vi "camara 2.vi"() -> ()   [LabVIEW 2010]
uses:
  <vilib>/addons/PixeLINK/Low Level Functions/CAMERA_FEATURES.llb/TDPU-CameraFeatures-PixelFormat.ctl
  <vilib>/addons/PixeLINK/Low Level Functions/ACQUISITION.llb/TDPU-Acquisition-StreamState.ctl
  <vilib>/addons/PixeLINK/Low Level Functions/CAMERA_FEATURES.llb/TDPU-CameraFeatures-FeatureIds.ctl
  <vilib>/addons/PixeLINK/Low Level Functions/CAMERA_FEATURES.llb/TDPU-CameraFeatures-FeatureFlags.ctl
panel:
  out "Data OUT":u8[](array[numeric])
  in  "Streeam":bool
  in  "Pixel Format Requerido":T1 items=["PIXEL_FORMAT_MONO8", "PIXEL_FORMAT_MONO16", "PIXEL_FORMAT_YUV422", "PIXEL_FORMAT_BAYER8_GRBG", "PIXEL_FORMAT_BAYER16_GRBG", "PIXEL_FORMAT_RGB24", "PIXEL_FORMAT_RGB48", "PIXEL_FORMAT_BAYER8_RGGB", "PIXEL_FORMAT_BAYER8_GBRG ", "PIXEL_FORMAT_BAYER8_BGGR ", "PIXEL_FORMAT_BAYER16_RGGB ", "PIXEL_FORMAT_BAYER16_GBRG", "PIXEL_FORMAT_BAYER16_BGGR", "PIXEL_FORMAT_RGB32"]
  out "Numeric":i32
  in  "Stop App":bool
  out "Numero de Camaras":u32
  in  "Selector":u16(ring) items=["776002034"]
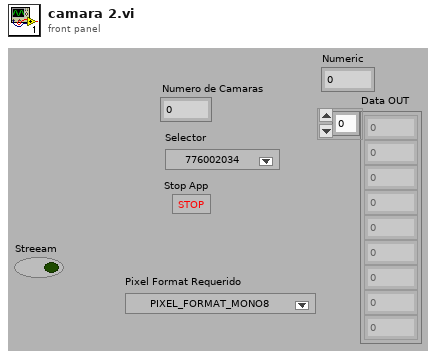
[diagram p1: front panel]
types:
  T1 = typedef "TDPU-CameraFeatures-PixelFormat.ctl" = u16
  T2 = typedef "TDPU-Acquisition-StreamState.ctl" = u32
  T3 = typedef "TDPU-CameraFeatures-FeatureIds.ctl" = u32
  T4 = typedef "TDPU-CameraFeatures-FeatureFlags.ctl" = u32
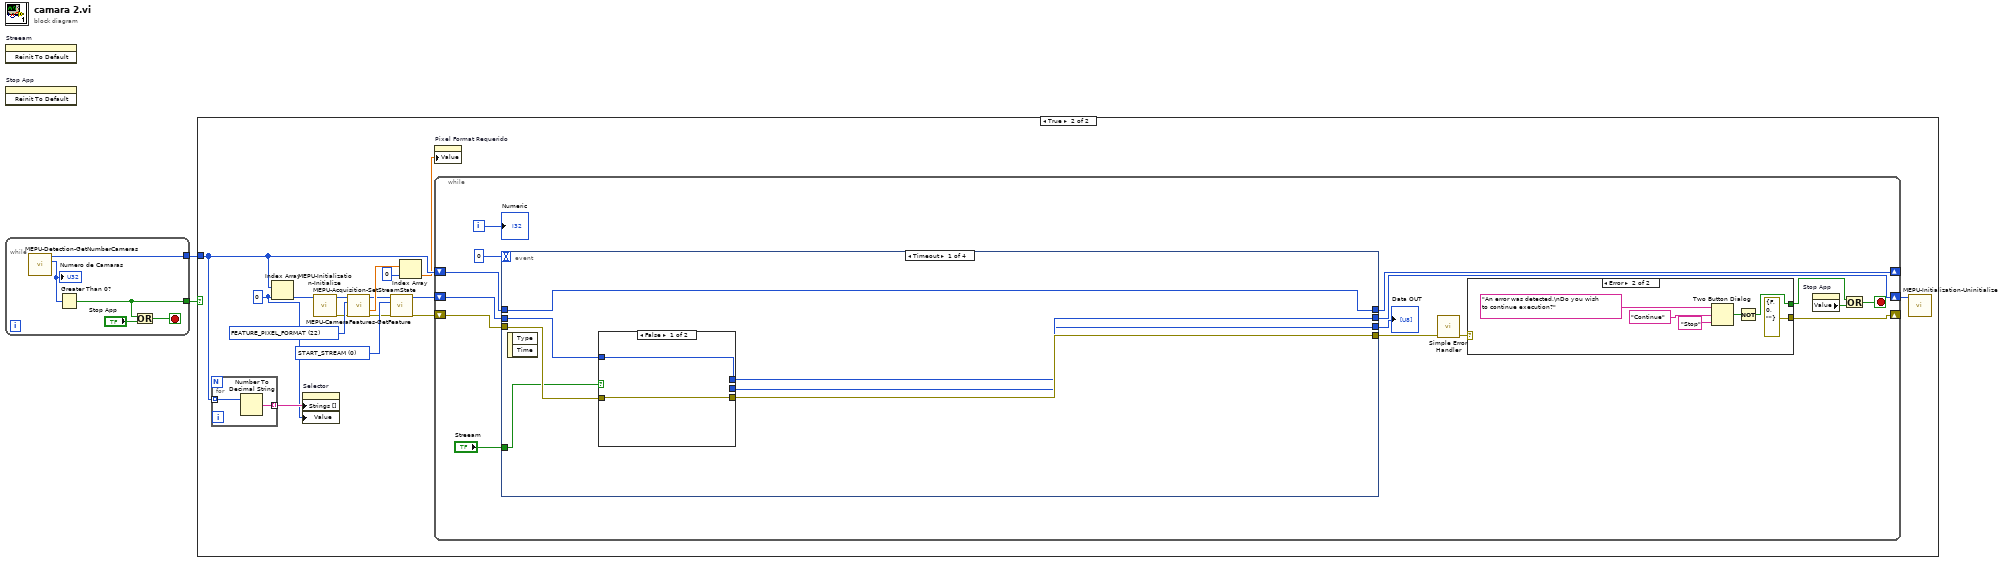
[diagram p0: block diagram]
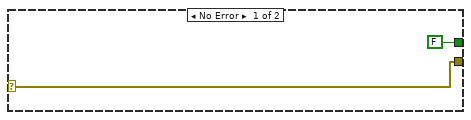
[diagram p3: hidden frame]
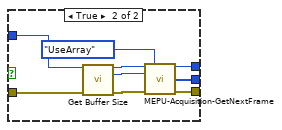
[diagram p4: hidden frame]
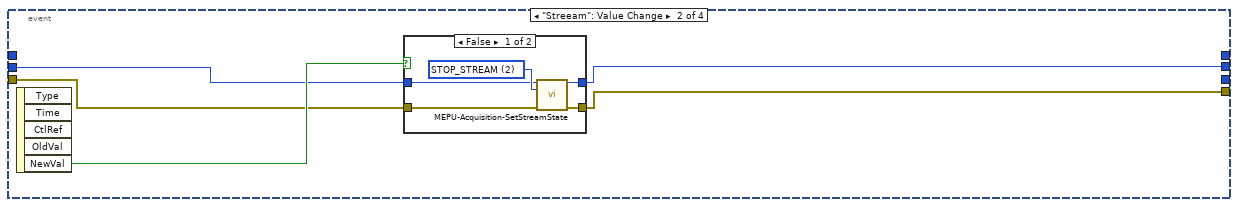
[diagram p5: hidden frame]
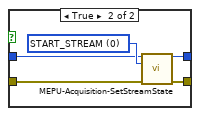
[diagram p6: hidden frame]
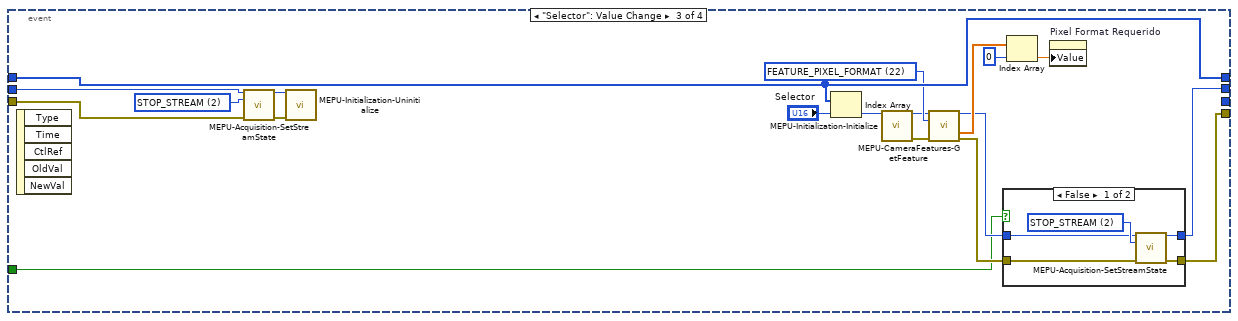
[diagram p7: hidden frame]
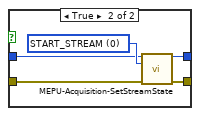
[diagram p8: hidden frame]
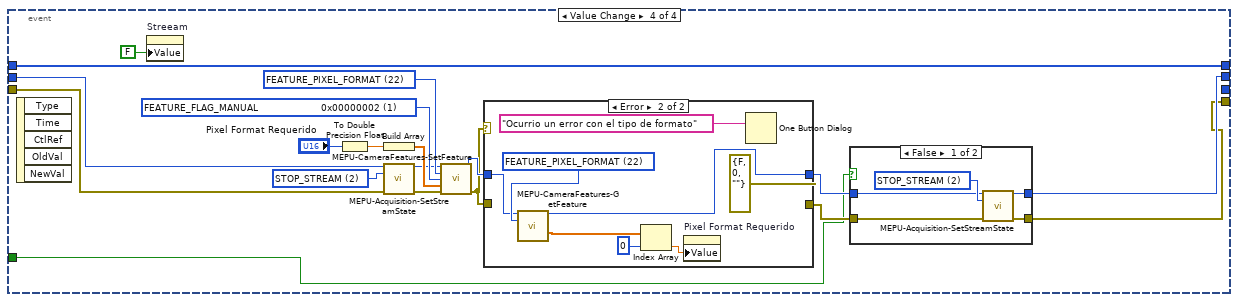
[diagram p9: hidden frame]
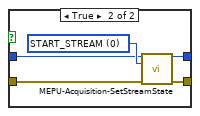
[diagram p10: hidden frame]
diagram:
  n1 = invoke on="Streeam" class="Bool (strict)" method="Reinit To Default"() -> ()  [unwired: 3 in, 3 out]
  n2 = invoke on="Stop App" class="Bool (strict)" method="Reinit To Default"() -> ()  [unwired: 3 in, 3 out]
  n3 = while {
    tunnel: [w7] -> w2
    tunnel: [w3] -> w1
    stop <- w5 stop-if-true
    n4 = call <vilib>:"MEPU-Detection-GetNumberCameras.vi"() -> ("LV_SerialNumbers OUT"=w7:u32[], "LV_NumberSerial OUT"=w4:u32)  [unwired: 13 in, 1 out]
    "Numero de Camaras" <- w4
    n5 = Greater Than 0?(x=w4) -> (x > 0?=w3:bool)
    n6 = Or(x=w3, y="Stop App") -> (x .or. y?=w5:bool)
  }
  n7 = case shown="True" w1 {
    tunnel: w2 -> [_ w21]
    frame False {
    }
    frame True {
      w12 = T2 0 items=["START_STREAM", "PAUSE_STREAM", "STOP_STREAM"] ("uStreamState IN")
      w17 = T3 22 items=["FEATURE_BRIGHTNESS", "FEATURE_EXPOSURE", "FEATURE_SHARPNESS", "FEATURE_WHITE_BAL", "FEATURE_HUE", "FEATURE_SATURATION", "FEATURE_GAMMA", "FEATURE_SHUTTER", "FEATURE_GAIN", "FEATURE_IRIS", "FEATURE_FOCUS", "FEATURE_TEMPERATURE", "FEATURE_TRIGGER", "FEATURE_ZOOM", "FEATURE_PAN", "FEATURE_TILT", "FEATURE_OPT_FILTER", "FEATURE_GPIO", "FEATURE_FRAME_RATE", "FEATURE_ROI", "FEATURE_FLIP", "FEATURE_PIXEL_ADDRESSING", "FEATURE_PIXEL_FORMAT", "FEATURE_EXTENDED_SHUTTER", "FEATURE_AUTO_ROI", "FEATURE_LOOKUP_TABLE", "FEATURE_MEMORY_CHANNEL", "FEATURE_WHITE_SHADING", "FEATURE_ROTATE", "FEATURE_IMAGER_CLK_DIVISOR", "FEATURE_TRIG_WITH_CNTRLD_LIGHT", "FEATURE_MAX_PIXEL_SIZE"] ("uFeatureId IN")
      w20 = 0
      n8 = for {
        tunnel: w21 -> [w149] mode=indexing
        tunnel: [w148] -> w23 mode=indexing
        n9 = Number To Decimal String(number=w149) -> (decimal integer string=w148:string)  [unwired: 1 in]
      }
      n10 = Index Array(array=w21, index=w20) -> (element=w22:u32)
      n11 = property on="Selector" class="Ring (strict)"("Strings []"=w23, "Value"=w20) -> ()  [unwired: 2 in, 2 out]
      n12 = call <vilib>:"MEPU-Initialization-Initialize.vi"("uSerialNumber IN"=w22) -> ("phCamera OUT"=w14:u32, "Error OUT"=w13:errorcluster)  [unwired: 12 in, 1 out]
      n13 = call <vilib>:"MEPU-CameraFeatures-GetFeature.vi"("hCamera IN"=w14, "uFeatureId IN"=w17, "Error IN"=w13) -> ("hCamera OUT"=w9:u32, "pParms OUT"=w18:dbl[], "Error OUT"=w10:errorcluster)  [unwired: 8 in, 2 out]
      n14 = call <vilib>:"MEPU-Acquisition-SetStreamState.vi"("hCamera IN"=w9, "uStreamState IN"=w12, "Error IN"=w10) -> ("hCamera OUT"=w8:u32, "Error OUT"=w11:errorcluster)  [unwired: 11 in]
      n15 = Index Array(array=w18, index=0) -> (element=w15:dbl)
      n16 = property on="Pixel Format Requerido" class="Ring (strict)"("Value"=w15) -> ()  [unwired: 2 in, 2 out]
      n17 = while {
        shift-right: [w37] -> _
        shift-left: w21 -> [w38]
        shift-right: [w26] -> w19
        shift-left: w8 -> [w36]
        shift-right: [w31] -> _
        shift-left: w11 -> [w35]
        i -> [w30]
        stop <- w32 stop-if-true
        n18 = event shown="[0] Timeout" {
          selector: _ -> [_ _ _ _]
          dyn-events: _ -> [_ _ _ _]
          timeout: 0 -> [_ _ _ _]
          tunnel: w38 -> [w53 _ w96 w114]
          tunnel: [w50 w66 w81 w113] -> w26
          tunnel: [w51 w65 w84 w112] -> w27
          tunnel: [w53 _ w96 w114] -> w37
          tunnel: w36 -> [w52 w68 w85 w120]
          tunnel: w35 -> [w48 w67 w86 w119]
          tunnel: [w49 _ _ _] -> w25
          tunnel: "Streeam" -> [w47 _ w80 w109]
          event Timeout {
            n19 = event-data() -> ()  [unwired: 1 in, 2 out]
            n20 = case shown="False" w47 {
              tunnel: w52 -> [w55 w60]
              tunnel: [w54 w59] -> w51
              tunnel: [w55 w58] -> w50
              tunnel: [_ w57] -> w49
              tunnel: w48 -> [w54 w56]
              frame False {
              }
              frame True {
                n21 = call "Get Buffer Size.vi"("phCamera IN"=w60, "Error IN"=w56) -> ("phCamera OUT"=w61:u32, "uBufferSize OUT"=w63:u32, "Error OUT"=w64:errorcluster)  [unwired: 11 out]
                n22 = call <vilib>:"MEPU-Acquisition-GetNextFrame.vi"("hCamera IN"=w61, "Mode IN"=enum16{"UseArray", "UsePointer"}."UseArray", "uBufferSize IN"=w63, "Error IN"=w64) -> ("hCamera OUT"=w58:u32, "Data OUT"=w57:u8[], "Error OUT"=w59:errorcluster)  [unwired: 7 in, 2 out]
              }
            }
          }
          event "Streeam": Value Change {
            n23 = event-data() -> ("NewVal"=w69:bool)  [unwired: 1 in, 4 out]
            n24 = case shown="False" w69 {
              tunnel: w68 -> [w73 w78]
              tunnel: w67 -> [w72 w77]
              tunnel: [w70 w76] -> w65
              tunnel: [w71 w75] -> w66
              frame False {
                w74 = T2 2 items=["START_STREAM", "PAUSE_STREAM", "STOP_STREAM"] ("uStreamState IN")
                n25 = call <vilib>:"MEPU-Acquisition-SetStreamState.vi"("hCamera IN"=w73, "uStreamState IN"=w74, "Error IN"=w72) -> ("hCamera OUT"=w71:u32, "Error OUT"=w70:errorcluster)  [unwired: 11 in]
              }
              frame True {
                w79 = T2 0 items=["START_STREAM", "PAUSE_STREAM", "STOP_STREAM"] ("uStreamState IN")
                n26 = call <vilib>:"MEPU-Acquisition-SetStreamState.vi"("hCamera IN"=w78, "uStreamState IN"=w79, "Error IN"=w77) -> ("hCamera OUT"=w75:u32, "Error OUT"=w76:errorcluster)  [unwired: 11 in]
              }
            }
          }
          event "Selector": Value Change {
            w89 = T2 2 items=["START_STREAM", "PAUSE_STREAM", "STOP_STREAM"] ("uStreamState IN")
            w95 = T3 22 items=["FEATURE_BRIGHTNESS", "FEATURE_EXPOSURE", "FEATURE_SHARPNESS", "FEATURE_WHITE_BAL", "FEATURE_HUE", "FEATURE_SATURATION", "FEATURE_GAMMA", "FEATURE_SHUTTER", "FEATURE_GAIN", "FEATURE_IRIS", "FEATURE_FOCUS", "FEATURE_TEMPERATURE", "FEATURE_TRIGGER", "FEATURE_ZOOM", "FEATURE_PAN", "FEATURE_TILT", "FEATURE_OPT_FILTER", "FEATURE_GPIO", "FEATURE_FRAME_RATE", "FEATURE_ROI", "FEATURE_FLIP", "FEATURE_PIXEL_ADDRESSING", "FEATURE_PIXEL_FORMAT", "FEATURE_EXTENDED_SHUTTER", "FEATURE_AUTO_ROI", "FEATURE_LOOKUP_TABLE", "FEATURE_MEMORY_CHANNEL", "FEATURE_WHITE_SHADING", "FEATURE_ROTATE", "FEATURE_IMAGER_CLK_DIVISOR", "FEATURE_TRIG_WITH_CNTRLD_LIGHT", "FEATURE_MAX_PIXEL_SIZE"] ("uFeatureId IN")
            n27 = event-data() -> ()  [unwired: 1 in, 5 out]
            n28 = call <vilib>:"MEPU-Acquisition-SetStreamState.vi"("hCamera IN"=w85, "uStreamState IN"=w89, "Error IN"=w86) -> ("hCamera OUT"=w87:u32, "Error OUT"=w88:errorcluster)  [unwired: 11 in]
            n29 = call <vilib>:"MEPU-Initialization-Uninitialize.vi"("hCamera IN"=w87, "Error IN"=w88) -> ()  [unwired: 13 in, 1 out]
            n30 = Index Array(array=w96, index="Selector") -> (element=w97:u32)
            n31 = call <vilib>:"MEPU-Initialization-Initialize.vi"("uSerialNumber IN"=w97) -> ("phCamera OUT"=w92:u32, "Error OUT"=w90:errorcluster)  [unwired: 12 in, 1 out]
            n32 = call <vilib>:"MEPU-CameraFeatures-GetFeature.vi"("hCamera IN"=w92, "uFeatureId IN"=w95, "Error IN"=w90) -> ("hCamera OUT"=w83:u32, "pParms OUT"=w94:dbl[], "Error OUT"=w82:errorcluster)  [unwired: 8 in, 2 out]
            n33 = case shown="False" w80 {
              tunnel: w83 -> [w102 w107]
              tunnel: w82 -> [w101 w106]
              tunnel: [w99 w105] -> w84
              tunnel: [w100 w104] -> w81
              frame False {
                w103 = T2 2 items=["START_STREAM", "PAUSE_STREAM", "STOP_STREAM"] ("uStreamState IN")
                n34 = call <vilib>:"MEPU-Acquisition-SetStreamState.vi"("hCamera IN"=w102, "uStreamState IN"=w103, "Error IN"=w101) -> ("hCamera OUT"=w100:u32, "Error OUT"=w99:errorcluster)  [unwired: 11 in]
              }
              frame True {
                w108 = T2 0 items=["START_STREAM", "PAUSE_STREAM", "STOP_STREAM"] ("uStreamState IN")
                n35 = call <vilib>:"MEPU-Acquisition-SetStreamState.vi"("hCamera IN"=w107, "uStreamState IN"=w108, "Error IN"=w106) -> ("hCamera OUT"=w104:u32, "Error OUT"=w105:errorcluster)  [unwired: 11 in]
              }
            }
            n36 = Index Array(array=w94, index=0) -> (element=w91:dbl)
            n37 = property on="Pixel Format Requerido" class="Ring (strict)"("Value"=w91) -> ()  [unwired: 2 in, 2 out]
          }
          event Value Change {
            w116 = T2 2 items=["START_STREAM", "PAUSE_STREAM", "STOP_STREAM"] ("uStreamState IN")
            w126 = T4 1 items=["FEATURE_FLAG_PRESENCE                 0x00000001", "FEATURE_FLAG_MANUAL                     0x00000002", "FEATURE_FLAG_AUTO                         0x00000004", "FEATURE_FLAG_ONEPUSH                   0x00000008", "FEATURE_FLAG_OFF                            0x00000010", "FEATURE_FLAG_DESC_SUPPORTED    0x00000020", "FEATURE_FLAG_READ_ONLY               0x00000040"] ("uFlags IN")
            w127 = T3 22 items=["FEATURE_BRIGHTNESS", "FEATURE_EXPOSURE", "FEATURE_SHARPNESS", "FEATURE_WHITE_BAL", "FEATURE_HUE", "FEATURE_SATURATION", "FEATURE_GAMMA", "FEATURE_SHUTTER", "FEATURE_GAIN", "FEATURE_IRIS", "FEATURE_FOCUS", "FEATURE_TEMPERATURE", "FEATURE_TRIGGER", "FEATURE_ZOOM", "FEATURE_PAN", "FEATURE_TILT", "FEATURE_OPT_FILTER", "FEATURE_GPIO", "FEATURE_FRAME_RATE", "FEATURE_ROI", "FEATURE_FLIP", "FEATURE_PIXEL_ADDRESSING", "FEATURE_PIXEL_FORMAT", "FEATURE_EXTENDED_SHUTTER", "FEATURE_AUTO_ROI", "FEATURE_LOOKUP_TABLE", "FEATURE_MEMORY_CHANNEL", "FEATURE_WHITE_SHADING", "FEATURE_ROTATE", "FEATURE_IMAGER_CLK_DIVISOR", "FEATURE_TRIG_WITH_CNTRLD_LIGHT", "FEATURE_MAX_PIXEL_SIZE"] ("uFeatureId IN")
            n38 = event-data() -> ()  [unwired: 1 in, 5 out]
            n39 = property on="Streeam" class="Bool (strict)"("Value"=FALSE ("Boolean")) -> ()  [unwired: 2 in, 2 out]
            n40 = To Double Precision Float(number="Pixel Format Requerido") -> (double precision float=w124:dbl)
            n41 = Build Array(w124) -> (w125:dbl[])
            n42 = call <vilib>:"MEPU-Acquisition-SetStreamState.vi"("hCamera IN"=w120, "uStreamState IN"=w116, "Error IN"=w119) -> ("hCamera OUT"=w118:u32, "Error OUT"=w117:errorcluster)  [unwired: 11 in]
            n43 = call <vilib>:"MEPU-CameraFeatures-SetFeature.vi"("hCamera IN"=w118, "uFeatureId IN"=w127, "uFlags IN"=w126, "pParms IN"=w125, "Error IN"=w117) -> ("hCamera OUT"=w122:u32, "Error OUT"=w121:errorcluster)  [unwired: 8 in, 1 out]
            n44 = case shown="Error" w121 {
              tunnel: w122 -> [w139 w144]
              tunnel: [w139 w143] -> w111
              tunnel: [w138 errorcluster {"status"=FALSE, "code"=0, "source"=""} ("Error OUT")] -> w110
              tunnel: w121 -> [w138 _]
              frame No Error {
              }
              frame Error {
                w147 = T3 22 items=["FEATURE_BRIGHTNESS", "FEATURE_EXPOSURE", "FEATURE_SHARPNESS", "FEATURE_WHITE_BAL", "FEATURE_HUE", "FEATURE_SATURATION", "FEATURE_GAMMA", "FEATURE_SHUTTER", "FEATURE_GAIN", "FEATURE_IRIS", "FEATURE_FOCUS", "FEATURE_TEMPERATURE", "FEATURE_TRIGGER", "FEATURE_ZOOM", "FEATURE_PAN", "FEATURE_TILT", "FEATURE_OPT_FILTER", "FEATURE_GPIO", "FEATURE_FRAME_RATE", "FEATURE_ROI", "FEATURE_FLIP", "FEATURE_PIXEL_ADDRESSING", "FEATURE_PIXEL_FORMAT", "FEATURE_EXTENDED_SHUTTER", "FEATURE_AUTO_ROI", "FEATURE_LOOKUP_TABLE", "FEATURE_MEMORY_CHANNEL", "FEATURE_WHITE_SHADING", "FEATURE_ROTATE", "FEATURE_IMAGER_CLK_DIVISOR", "FEATURE_TRIG_WITH_CNTRLD_LIGHT", "FEATURE_MAX_PIXEL_SIZE"] ("uFeatureId IN")
                n45 = call <vilib>:"MEPU-CameraFeatures-GetFeature.vi"("hCamera IN"=w144, "uFeatureId IN"=w147) -> ("hCamera OUT"=w143:u32, "pParms OUT"=w146:dbl[])  [unwired: 9 in, 3 out]
                n46 = Index Array(array=w146, index=0) -> (element=w141:dbl)
                n47 = property on="Pixel Format Requerido" class="Ring (strict)"("Value"=w141) -> ()  [unwired: 2 in, 2 out]
                n48 = One Button Dialog(message="Ocurrio un error con el tipo de formato") -> ()  [unwired: 1 in, 1 out]
              }
            }
            n49 = case shown="False" w109 {
              tunnel: w111 -> [w131 w136]
              tunnel: w110 -> [w130 w135]
              tunnel: [w128 w134] -> w112
              tunnel: [w129 w133] -> w113
              frame False {
                w132 = T2 2 items=["START_STREAM", "PAUSE_STREAM", "STOP_STREAM"] ("uStreamState IN")
                n50 = call <vilib>:"MEPU-Acquisition-SetStreamState.vi"("hCamera IN"=w131, "uStreamState IN"=w132, "Error IN"=w130) -> ("hCamera OUT"=w129:u32, "Error OUT"=w128:errorcluster)  [unwired: 11 in]
              }
              frame True {
                w137 = T2 0 items=["START_STREAM", "PAUSE_STREAM", "STOP_STREAM"] ("uStreamState IN")
                n51 = call <vilib>:"MEPU-Acquisition-SetStreamState.vi"("hCamera IN"=w136, "uStreamState IN"=w137, "Error IN"=w135) -> ("hCamera OUT"=w133:u32, "Error OUT"=w134:errorcluster)  [unwired: 11 in]
              }
            }
          }
        }
        "Data OUT" <- w25
        n52 = call <vilib>:"Simple Error Handler.vi"("error in (no error)"=w27) -> ("error out"=w34:errorcluster)  [unwired: 1 in, 7 out]
        n53 = case shown="Error" w34 {
          selector: w34 -> [w40 _]
          tunnel: [w40 errorcluster {"status"=FALSE, "code"=0, "source"=""} ("error IO")] -> w31
          tunnel: [FALSE ("T button?") w41] -> w33
          frame No Error {
          }
          frame Error {
            n54 = Two Button Dialog(message="An error was detected.\nDo you wish to continue execution?", 1:"Stop" ("F button name (\"Cancel\")"), 2:"Continue" ("T button name (\"OK\")")) -> (T button?=w42:bool)
            n55 = Not(x=w42) -> (.not. x?=w41:bool)
          }
        }
        n56 = property on="Stop App" class="Bool (strict)"() -> ("Value"=w28:bool)  [unwired: 2 in, 2 out]
        n57 = Or(x=w33, y=w28) -> (x .or. y?=w32:bool)
        "Numeric" <- w30
      }
      n58 = call <vilib>:"MEPU-Initialization-Uninitialize.vi"("hCamera IN"=w19) -> ()  [unwired: 14 in, 1 out]
    }
  }
